vi "Tosca-Initialize State.vi"(7 "Config":string, 11 "Error In":errorcluster) -> (4 "State":T1, 15 "error out":errorcluster)   [LabVIEW 2020]
uses:
  Typedefs/Tosca-State.ctl
  Typedefs/Tosca-Thread Type.ctl
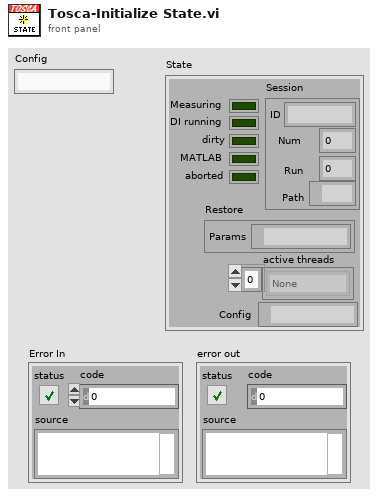
[diagram p1: front panel]
types:
  T1 = typedef "Tosca-State.ctl" = cluster{"Measuring":bool, "DI running":bool, "dirty":bool, "Restore":cluster{"Params":path}, "Session":cluster{"ID":string, "Num":i32, "Path":path, "Run":i32}, "active threads":T2[], "MATLAB":bool, "Config":path, "aborted":bool}
  T2 = typedef "Tosca-Thread Type.ctl" = enum16{"None", "AODO", "Masker", "ET", "Imaging", "Pupil", "AI", "DI", "Camera", "TTL out", "Loco", "Visual"}
  T3 = cluster{"ID":string, "Num":i32, "Path":path, "Run":i32}
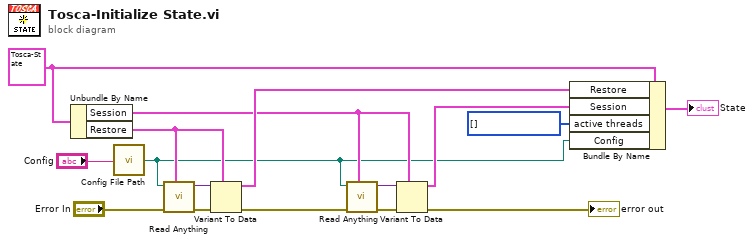
[diagram p0: block diagram]
diagram:
  w3 = T2[] [] items=["None", "AODO", "Masker", "ET", "Imaging", "Pupil", "AI", "DI", "Camera", "TTL out", "Loco", "Visual"] ("active threads")
  w8 = T1 {"Measuring"=FALSE, "DI running"=FALSE, "dirty"=FALSE, "Restore"={"Params"=path ""}, "Session"={"ID"="", "Num"=0, "Path"=path "", "Run"=0}, "active threads"=[], "MATLAB"=FALSE, "Config"=path "", "aborted"=FALSE} ("State")
  n1 = Unbundle By Name(w8) -> ("Session"=w6:T3, "Restore"=w9:cluster{"Params":path})
  n2 = call "Config File Path.vi"("AppName"="Config") -> ("Default config file name"=w1:path)
  n3 = call "Read Anything.vi"("Type of Anything"=w9, "Error In"="Error In", "Path (dialog)"=w1) -> ("Error Out"=w14:errorcluster, "Anything"=w16:variant)  [unwired: 6 in, 1 out]
  n4 = Variant To Data(error in=w14, type=w9, Variant=w16) -> (data=w7:cluster{"Params":path}, error out=w13:errorcluster)
  n5 = call "Read Anything.vi"("Type of Anything"=w6, "Error In"=w13, "Path (dialog)"=w1) -> ("Error Out"=w12:errorcluster, "Anything"=w15:variant)  [unwired: 6 in, 1 out]
  n6 = Variant To Data(error in=w12, type=w6, Variant=w15) -> (data=w5:T3, error out=→"error out":errorcluster)
  n7 = Bundle By Name(cluster=w8, "Restore"=w7, "Session"=w5, "active threads"=w3, "Config"=w1) -> (→"State":T1)
